vi "Create Sweep Settings Data.vi"(7 "DUT Name":string, 8 "error in (no error)":errorcluster, 10 "Sweep Points":cluster{"Pin":string, "Sweep Point":T1}[](array[cluster]) {"Sweep Point"."Frequency" format="%#_6p"}, 11 "Sweep Type":T2) -> (0 "error out":errorcluster, 2 "Sweep Settings Data":T3[](array[typedef]) {"Sweep Points"."Frequency" format="%#_6p"})   [LabVIEW 2016]
uses:
  RFPM CLB Calibration/RFPM CLB Calibration UI.lvlibp/Actors/RFPM CLB Calibration UI/RFPM CLB Calibration UI/TypeDefs/Sweep Points.ctl
  RFPM CLB Calibration/RFPM CLB Calibration UI.lvlibp/Actors/RFPM CLB Calibration UI/RFPM CLB Calibration UI/TypeDefs/Sweep Editor Data.ctl
  RFPM CLB Calibration/RFPM CLB Calibration UI.lvlibp/Actors/RFPM CLB Calibration Process/RFPM CLB Calibration Process/TypeDefs/Sweep Type.ctl
  RFPM CLB Calibration/RFPM CLB Calibration Process.lvlibp/RFPM CLB Calibration Process/TypeDefs/Sweep Type.ctl
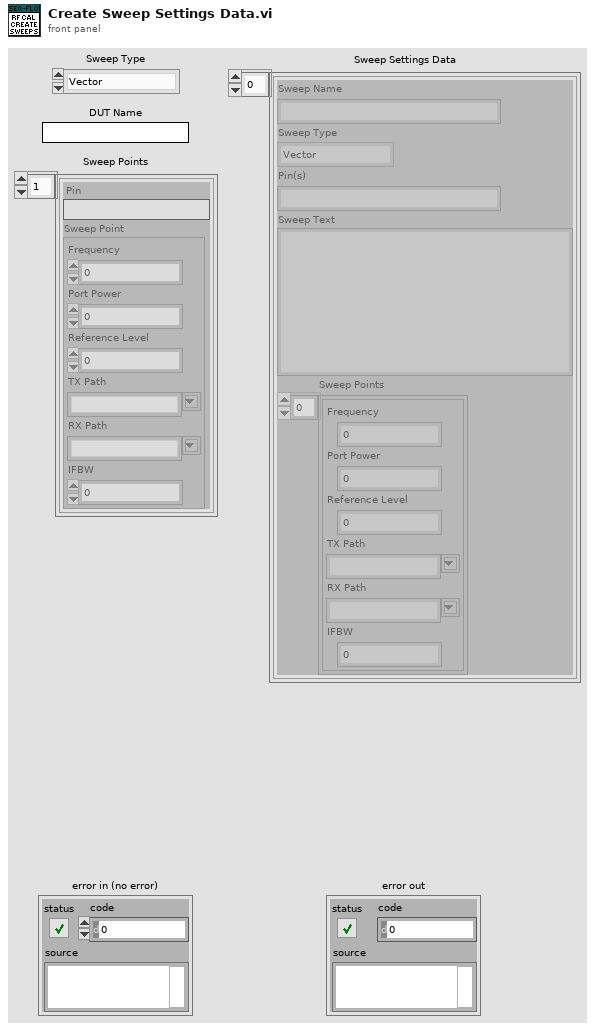
[diagram p1: front panel]
types:
  T1 = typedef "RFPM CLB Calibration UI.lvlibp/RFPM CLB Calibration UI.lvclass/Sweep Points.ctl" = cluster{"Frequency":dbl, "Port Power":dbl, "Reference Level":dbl, "TX Path":string, "RX Path":string, "IFBW":dbl}
  T2 = typedef "RFPM CLB Calibration Process.lvlibp/RFPM CLB Calibration Process.lvclass/Sweep Type.ctl" = enum16{"Vector", "Source", "Receiver"}
  T3 = typedef "RFPM CLB Calibration UI.lvlibp/RFPM CLB Calibration UI.lvclass/Sweep Editor Data.ctl" = cluster{"Sweep Name":string, "Sweep Type":T4, "Pin(s)":string, "Sweep Text":string, "Sweep Points":T1[]}
  T4 = typedef "RFPM CLB Calibration UI.lvlibp/RFPM CLB Calibration Process.lvlib/RFPM CLB Calibration Process.lvclass/Sweep Type.ctl" = enum16{"Vector", "Source", "Receiver"}
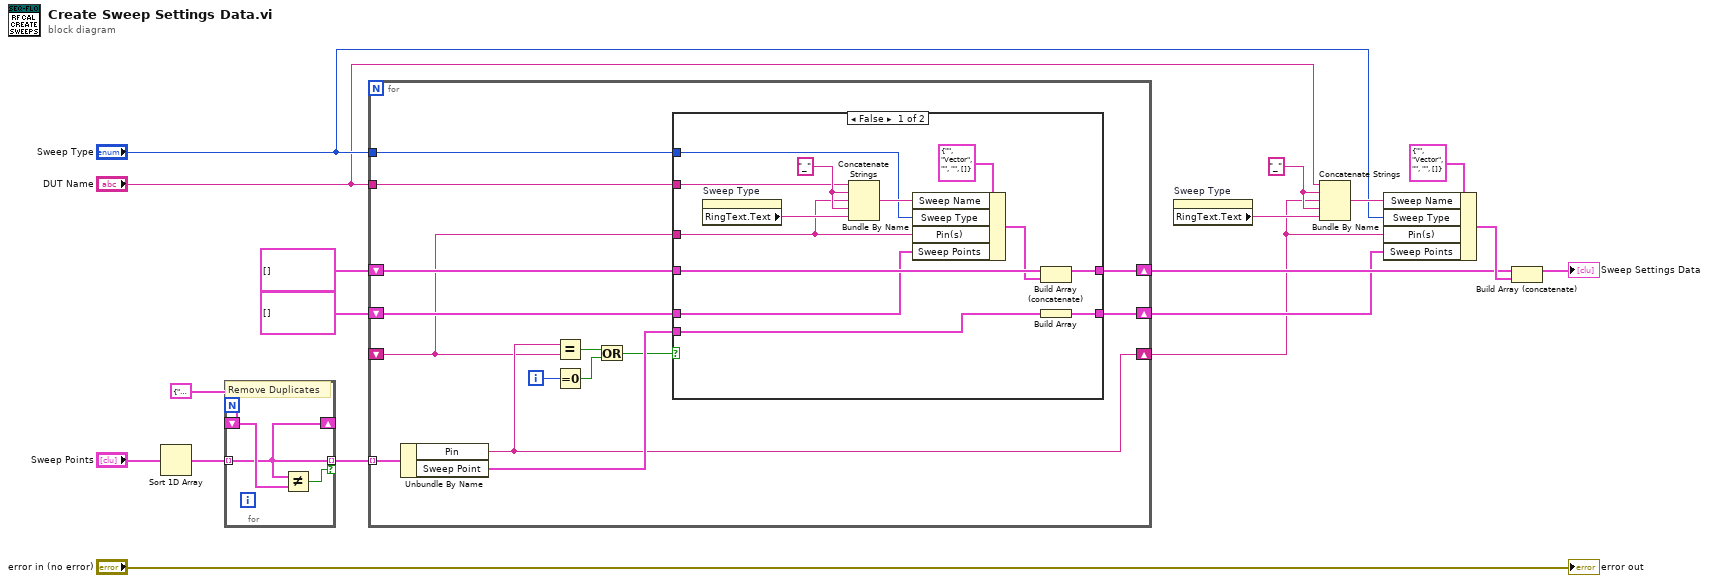
[diagram p0: block diagram]
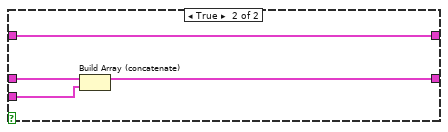
[diagram p2: hidden frame]
diagram:
  w9 = "_"
  n1 = Sort 1D Array(array="Sweep Points") -> (sorted array=w17:cluster{"Pin":string, "Sweep Point":T1}[])
  n2 = for {
    tunnel: [w20] -> w15 mode=indexing if=w19
    tunnel: w17 -> [w20] mode=indexing
    shift-right: [w20] -> _
    shift-left: cluster{"SG Pin":string, "Sweep Point":T1} {"SG Pin"="", "Sweep Point"={"Frequency"=0.0, "Port Power"=0.0, "Reference Level"=0.0, "TX Path"="", "RX Path"="", "IFBW"=0.0}} -> [w21]
    # "Remove Duplicates"
    n3 = Not Equal?(x=w20, y=w21) -> (x != y?=w19:bool)
  }
  n4 = for {
    tunnel: w15 -> [w35] mode=indexing
    shift-right: [w27] -> w1
    shift-left: _ -> [w22]
    shift-right: [w33] -> w6
    shift-left: T3[] [] -> [w34]
    shift-right: [w32] -> w2
    shift-left: T1[] [] ("Array in") -> [w30]
    tunnel: "Sweep Type" -> [w29]
    tunnel: "DUT Name" -> [w28]
    i -> [w26]
    n5 = Unbundle By Name(w35) -> ("Pin"=w27:string, "Sweep Point"=w31:T1)
    n6 = Equal?(x=w27, y=w22) -> (x = y?=w24:bool)
    n7 = Equal To 0?(x=w26) -> (x = 0?=w23:bool)
    n8 = Or(x=w24, y=w23) -> (x .or. y?=w25:bool)
    n9 = case shown="False" w25 {
      tunnel: w34 -> [w48 w52]
      tunnel: [w38 w52] -> w33
      tunnel: [w47 w50] -> w32
      tunnel: w31 -> [w40 w49]
      tunnel: w30 -> [w37 w51]
      tunnel: w29 -> [w42 _]
      tunnel: w28 -> [w41 _]
      tunnel: w22 -> [w36 _]
      frame False {
        w44 = "_"
        n10 = property on="Sweep Type" class="Enum (strict)"() -> ("RingText.Text"=w46:string)  [unwired: 2 in, 2 out]
        n11 = Concatenate Strings(w41, w44, w36, w44, w46) -> (w45:string)
        n12 = Bundle By Name(cluster=T3 {"Sweep Name"="", "Sweep Type"=enum."Vector", "Pin(s)"="", "Sweep Text"="", "Sweep Points"=[]} ("Sweep"), "Sweep Name"=w45, "Sweep Type"=w42, "Pin(s)"=w36, "Sweep Points"=w37) -> (w39:T3)
        n13 = Build Array (concatenate)(w48, w39) -> (w38:T3[])
        n14 = Build Array(w40) -> (w47:T1[])
      }
      frame True {
        n15 = Build Array (concatenate)(w51, w49) -> (w50:T1[])
      }
    }
  }
  n16 = property on="Sweep Type" class="Enum (strict)"() -> ("RingText.Text"=w7:string)  [unwired: 2 in, 2 out]
  n17 = Concatenate Strings("DUT Name", w9, w1, w9, w7) -> (w8:string)
  n18 = Bundle By Name(cluster=T3 {"Sweep Name"="", "Sweep Type"=enum."Vector", "Pin(s)"="", "Sweep Text"="", "Sweep Points"=[]} ("Sweep"), "Sweep Name"=w8, "Sweep Type"="Sweep Type", "Pin(s)"=w1, "Sweep Points"=w2) -> (w11:T3)
  n19 = Build Array (concatenate)(w6, w11) -> (→"Sweep Settings Data":T3[])
  "error out" <- "error in (no error)"
